vi "Replace Spaces by Web-safe Equivalent.vi"(2 "String in":string) -> (7 "String out":string)   [LabVIEW 2021, in "Strings.lvlib"]
uses:
  Strings.lvlib
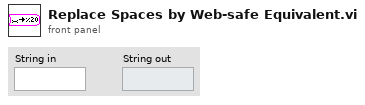
[diagram p1: front panel]
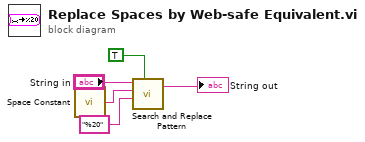
[diagram p0: block diagram]
diagram:
  n1 = call <vilib>:"Space Constant.vi"() -> ("String"=w4:string)
  n2 = call <vilib>:"Search and Replace Pattern.vi"("string"="String in", "regular expression (\"\")"=w4, "replace string (\"\")"="%20" ("replace string (\"\")"), "replace all? (F)"=TRUE) -> ("result string"=→"String out":string)  [unwired: 1 in, 1 out]
